vi "Sigma_MoveXY.vi"(7 "Travel per Pulse (0.004mm)":dbl=0.004, 8 "error in (no error)":errorcluster, 9 "Travel Axis 2 (mm)":dbl=1.0 format="%#_2f", 10 "Travel Axis 1 (mm)":dbl=1.0 format="%#_2f", 11 "VISA resource name":refnum<visa-resource-name>) -> (0 "error out":errorcluster, 3 "VISA resource name out":refnum<visa-resource-name>)   [LabVIEW 2012]
panel:
  out "결과 문자열":string
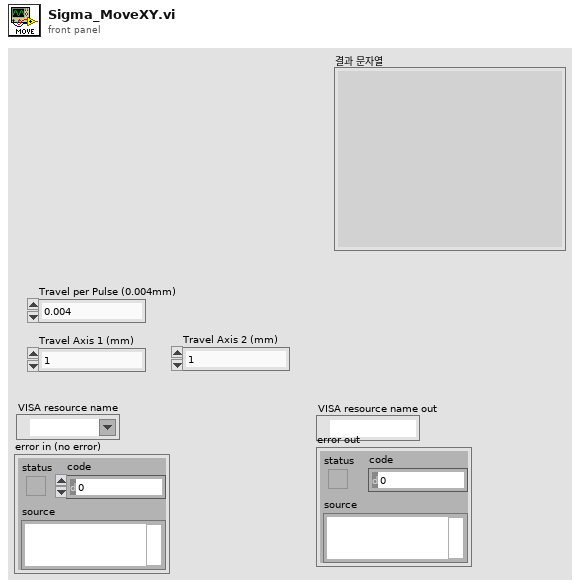
[diagram p1: front panel]
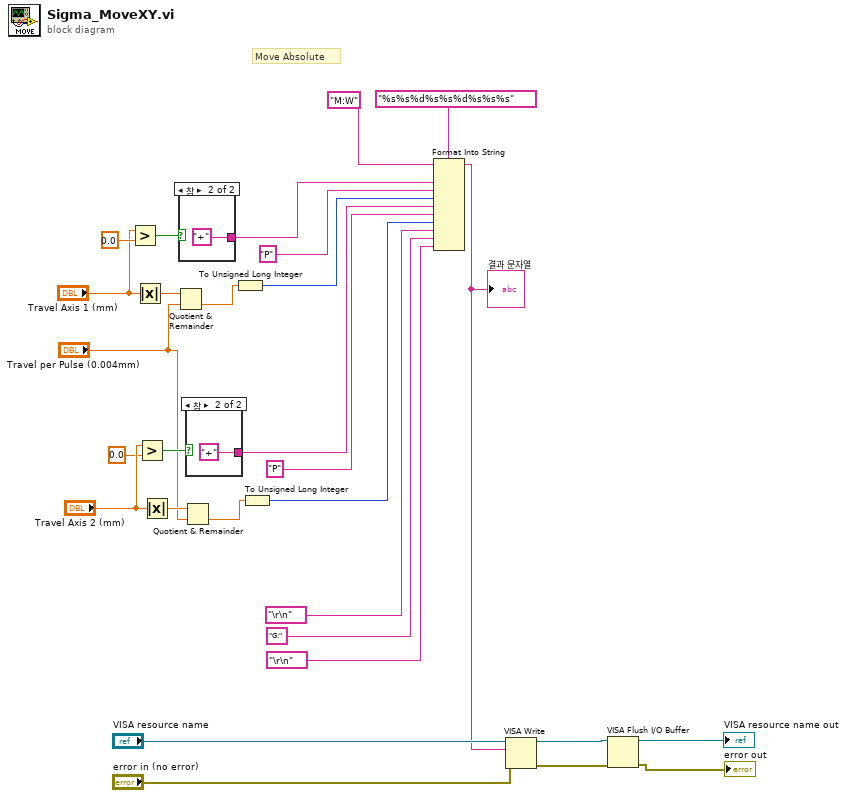
[diagram p0: block diagram]
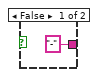
[diagram p2: hidden frame]
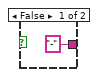
[diagram p3: hidden frame]
diagram:
  # "Move Absolute"
  n1 = Greater?(x="Travel Axis 1 (mm)", y=0.0) -> (0:w13:bool)
  n2 = Absolute Value(x="Travel Axis 1 (mm)") -> (abs(x)=w10:dbl)
  n3 = Greater?(x="Travel Axis 2 (mm)", y=0.0) -> (0:w6:bool)
  n4 = Absolute Value(x="Travel Axis 2 (mm)") -> (abs(x)=w9:dbl)
  n5 = Quotient & Remainder(x=w10, y="Travel per Pulse (0.004mm)") -> (floor(x/y)=w15:dbl)  [unwired: 1 out]
  n6 = case shown="참" w13 {
    tunnel: ["-" "+"] -> w25
    frame False {
    }
    frame True {
    }
  }
  n7 = Quotient & Remainder(x=w9, y="Travel per Pulse (0.004mm)") -> (floor(x/y)=w5:dbl)  [unwired: 1 out]
  n8 = case shown="참" w6 {
    tunnel: ["-" "+"] -> w3
    frame False {
    }
    frame True {
    }
  }
  n9 = To Unsigned Long Integer(number=w15) -> (unsigned 32bit integer=w14:u32)
  n10 = To Unsigned Long Integer(number=w5) -> (unsigned 32bit integer=w4:u32)
  n11 = Format Into String(format string="%s%s%d%s%s%d%s%s%s", initial string="M:W" ("string"), w25, "P" ("input 3"), w14, w3, "P" ("input 3"), w4, "\r\n" ("input 3"), "G:" ("input 3"), "\r\n" ("input 3")) -> (resulting string=w22:string)  [unwired: 1 in, 1 out]
  "결과 문자열" <- w22
  n12 = VISA Write(VISA resource name="VISA resource name", write buffer=w22, error in (no error)="error in (no error)") -> (VISA resource name out=w19:refnum<visa-resource-name>, error out=w18:errorcluster)  [unwired: 1 out]
  n13 = VISA Flush I/O Buffer(VISA resource name=w19, error in (no error)=w18) -> (VISA resource name out=→"VISA resource name out":refnum<visa-resource-name>, error out=→"error out":errorcluster)  [unwired: 1 in]
